vi "Init.vi"(7 "Section Name":refnum<class "Section Name.lvclass">, 8 "Error In":errorcluster, 9 "Values":refnum<class "Value.lvclass">[](array[class]), 10 "Keys":refnum<class "Key Name.lvclass">[](array[class]), 11 "reference in":refnum<class "OD Entry.lvclass">) -> (0 "Error Out":errorcluster, 3 "reference out":refnum<class "OD Entry.lvclass">)   [LabVIEW 2024, in "Electronic Datasheet.lvlib" / "OD Entry.lvclass"]
doc: "Indices in the EDS are always in hex format without the pre 0x"
uses:
  OD Entry.lvclass
  Keyname/Key Name.lvclass
  Value/Value.lvclass
  Section Name/Section Name.lvclass
  DOMAIN/DOMAIN.lvclass
  VAR/VAR.lvclass
  ARRAY/ARRAY.lvclass
  RECORD/RECORD.lvclass
  Object Type/Object Type Base.lvclass
  OD Entry.lvclass/OD Entry.ctl
  Object Type.ctl
  Electronic Datasheet.lvlib
  PDO Mapping Type.ctl
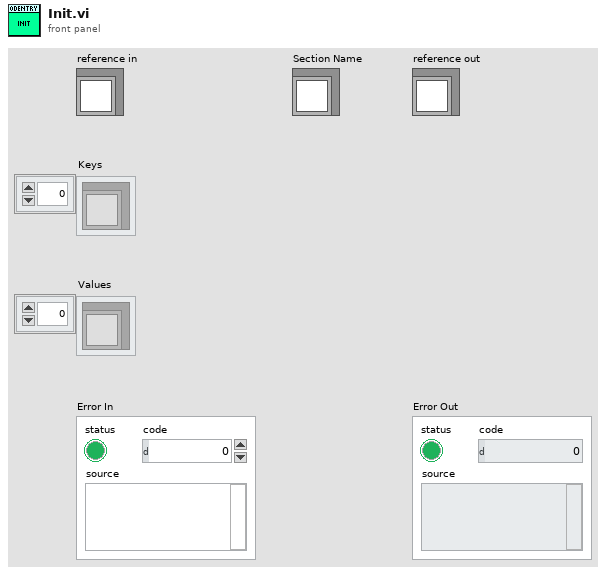
[diagram p1: front panel]
types:
  T1 = typedef "Electronic Datasheet.lvlib/PDO Mapping Type.ctl" = enum16{"no", "optional", "RPDO", "TPDO", "UNKNOWN"}
  T2 = typedef "Electronic Datasheet.lvlib/Object Type.ctl" = u8
  T3 = typedef "Electronic Datasheet.lvlib/OD Entry.lvclass/ObjectAttributes.ctl" = cluster{"Index":u16, "ObjectType":refnum<class "Object Type Base.lvclass">, "Denotation":string, "Count":u8, "ObjExtend":u8, "Label":string, "Description":string, "PDO Mapping Type":T1, "Sub-Entries":map{u8, refnum<class "OD Sub-Entry.lvclass">}}
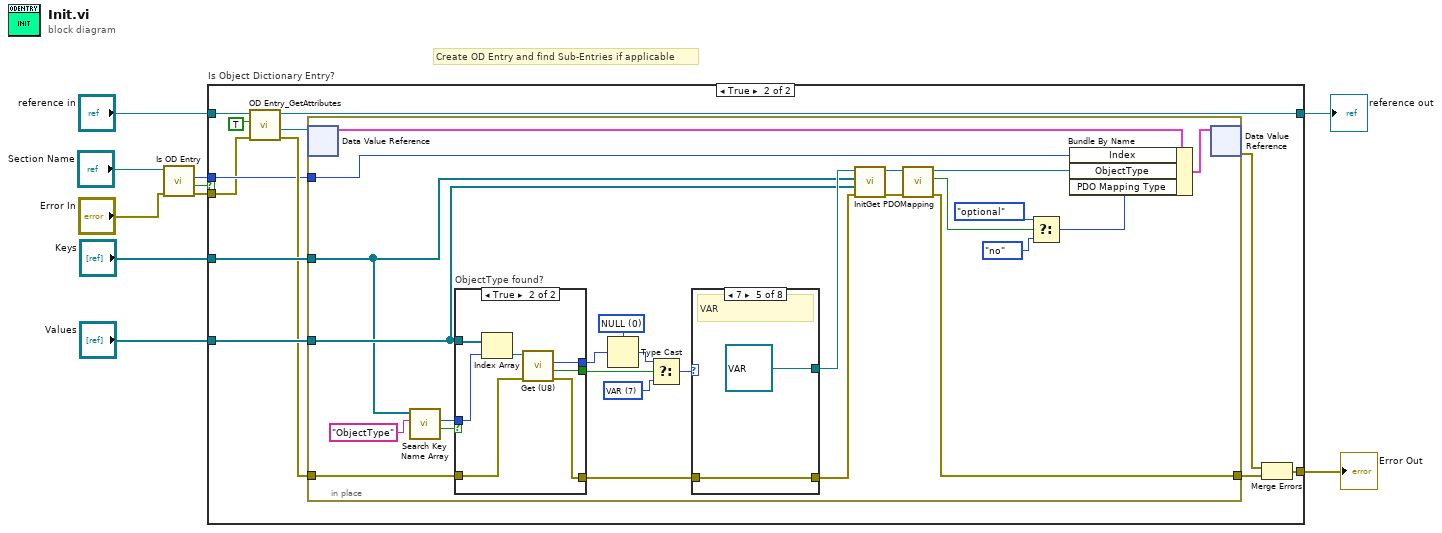
[diagram p0: block diagram]
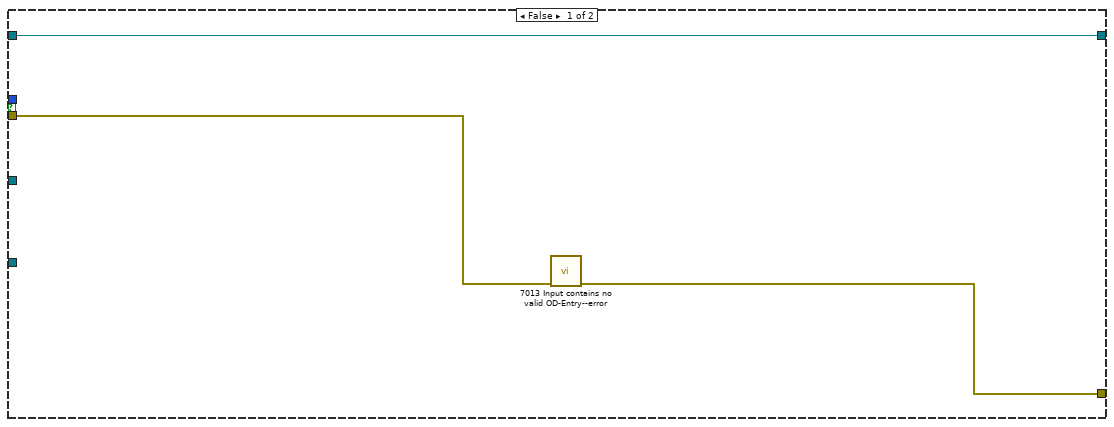
[diagram p2: hidden frame]
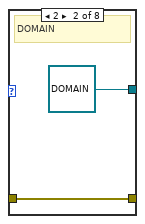
[diagram p4: hidden frame]
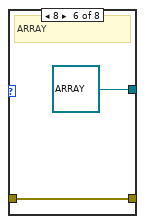
[diagram p7: hidden frame]
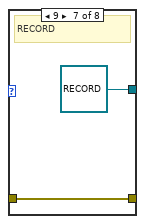
[diagram p8: hidden frame]
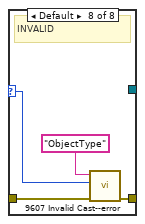
[diagram p9: hidden frame]
diagram:
  # "Create OD Entry and find Sub-Entries if applicable"
  n1 = call "Is OD Entry.vi"("error in"="Error In", "Section Name in"="Section Name") -> ("error out"=w2:errorcluster, "Is OD Entry?"=w1:bool, "Index"=w5:u16)  [unwired: 5 in, 2 out]
  n2 = case "Is Object Dictionary Entry?" shown="True" w1 {
    tunnel: [w11 w25] -> w10
    tunnel: [w13 w24] -> w9
    tunnel: "Keys" -> [_ w23]
    tunnel: "Values" -> [_ w22]
    tunnel: "reference in" -> [w13 w18]
    tunnel: w5 -> [_ w15]
    tunnel: w2 -> [w12 w14]
    frame False {
      n3 = call "7013 Input contains no valid OD-Entry--error.vi"("error in"=w12) -> ("error out"=w11:errorcluster)  [unwired: 10 in]
    }
    frame True {
      n4 = call "OD Entry_GetAttributes.vi"("Error In"=w14, "OnlyGetDvrReference(False)"=TRUE, "reference in"=w18) -> ("Error Out"=w17:errorcluster, "DataRef"=w19:refnum<data-value>, "reference out"=w24:refnum<class "OD Entry.lvclass">)  [unwired: 5 in, 1 out]
      n5 = in-place {
        in-place-border: w23 -> [w36]
        in-place-border: w22 -> [w37]
        in-place-border: w17 -> [w39]
        in-place-border: [w31] -> w16
        in-place-border: w15 -> [w34]
        w46 = T2 0 items=["NULL"=0, "DOMAIN"=2, "DEFTYPE"=5, "DEFSTRUCT"=6, "VAR"=7, "ARRAY"=8, "RECORD"=9] ("ObjectType")
        w42 = T2 7 items=["NULL"=0, "DOMAIN"=2, "DEFTYPE"=5, "DEFSTRUCT"=6, "VAR"=7, "ARRAY"=8, "RECORD"=9] ("ObjectType")
        n6 = in-place-dvr #1(w19) -> (w51:T3)  [unwired: 1 out]
        n7 = call "Search Key Name Array.vi"("Key Name"="ObjectType" ("String"), "Keys"=w36) -> ("Found?"=w48:bool, "Index"=w47:i32)  [unwired: 7 in, 1 out]
        n8 = case "ObjectType found?" shown="True" w48 {
          selector: w48 -> [w68 _]
          tunnel: w47 -> [_ w74]
          tunnel: w37 -> [_ w75]
          tunnel: w39 -> [w67 w72]
          tunnel: [w68 w71] -> w45
          tunnel: [_ w70] -> w44
          tunnel: [w67 w69] -> w40
          frame False {
          }
          frame True {
            n9 = Index Array(array=w75, index=w74) -> (element=w73:refnum<class "Value.lvclass">)
            n10 = call "Get (U8).vi"("error in"=w72, "Value in"=w73) -> ("error out"=w69:errorcluster, "Defined?"=w71:bool, "Value"=w70:u8)  [unwired: 6 in, 1 out]
          }
        }
        n11 = Type Cast(type=w46, x=w44) -> (*(type *) &x=w43:T2)
        n12 = Select(t=w43, s=w45, f=w42) -> (s? t:f=w41:T2)
        n13 = case shown="7" w41 {
          selector: w41 -> [_ _ _ _ _ _ _ w63]
          tunnel: w40 -> [w52 w54 w55 w56 w58 w59 w62 w66]
          tunnel: [w52 w54 w55 w56 w58 w59 w62 w64] -> w35
          tunnel: [_ refnum<class "DOMAIN.lvclass"> refnum ("EDS.lvlib:DOMAIN.lvclass") _ _ refnum<class "VAR.lvclass"> refnum ("EDS.lvlib:VAR.lvclass") refnum<class "ARRAY.lvclass"> refnum ("EDS.lvlib:ARRAY.lvclass") refnum<class "RECORD.lvclass"> refnum ("EDS.lvlib:RECORD.lvclass") _] -> w38
          frame 0 {
            # "NULL"
          }
          frame 2 {
            # "DOMAIN"
          }
          frame 5 {
            # "DEFTYPE"
          }
          frame 6 {
            # "DEFSTRUCT"
          }
          frame 7 {
            # "VAR"
          }
          frame 8 {
            # "ARRAY"
          }
          frame 9 {
            # "RECORD"
          }
          frame Default {
            # "INVALID"
            n14 = call "9607 Invalid Cast--error.vi"("error in"=w66, "Value"=w63, "Type"="ObjectType" ("error message (\"\")")) -> ("error out"=w64:errorcluster)  [unwired: 8 in]
          }
        }
        n15 = call-dynamic "Init.vi"("error in"=w35, "Values"=w37, "Keys"=w36, "Object Type in"=w38) -> ("error out"=w32:errorcluster, "Object Type out"=w33:refnum<class "Object Type Base.lvclass">)  [unwired: 6 in]
        n16 = call-dynamic "Get PDOMapping.vi"("error in"=w32, "Object Type in"=w33) -> ("error out"=w31:errorcluster, "PDOMapping"=w30:bool, "Object Type out"=w26:refnum<class "Object Type Base.lvclass">)  [unwired: 6 in, 1 out]
        n17 = Select(t=PDO_Mapping_Type."optional", s=w30, f=PDO_Mapping_Type."no" ("PDO Mapping Type")) -> (s? t:f=w27:T1)
        n18 = Bundle By Name(cluster=w51, "Index"=w34, "ObjectType"=w26, "PDO Mapping Type"=w27) -> (w50:T3)
        n19 = in-place-dvr #1(w50) -> (w20:errorcluster)  [unwired: 1 out]
      }
      n20 = Merge Errors(w20, w16) -> (w25:errorcluster)
    }
  }
  "Error Out" <- w10
  "reference out" <- w9
